vi "test.vi"() -> ()   [LabVIEW 2014]
panel:
  in  "id 4":string="R-6"
  in  "new_setting 4":dbl=0.2
  in  "id 3":string="R-6"
  in  "new_setting 3":dbl=1.0
  in  "new_setting 2":dbl=1.0
  in  "id 2":string="R-5"
  in  "new_setting":dbl=0.2
  in  "id":string="R-5"
  in  "Attribute 3":i32(ring)=201 items=["Depth"=200, "Volume"=201, "Flow"=202, "Setting"=203, "Froude"=204, "Inflow"=205, "Flooding"=206, "Precipitation"=207, "Runoff"=208]
  in  "Unit system 3":i32(ring)=1 items=["US", "SI"]
  in  "object_id 3":string="V-3"
  in  "object_id 2":string="V-2"
  in  "Attribute 2":i32(ring)=201 items=["Depth"=200, "Volume"=201, "Flow"=202, "Setting"=203, "Froude"=204, "Inflow"=205, "Flooding"=206, "Precipitation"=207, "Runoff"=208]
  in  "Unit system 2":i32(ring)=1 items=["US", "SI"]
  out "Graph":dbl[][](graph)
  in  "Path":path=path "C:/Users/andres riaño/Dropbox/Proyecto Aguas/Software/MatSWMM/MatSWMM 5.1.009/LabVIEW module/x64/swmm_files/3tanks.INP"
  in  "Unit system":i32(ring)=1 items=["US", "SI"]
  in  "Attribute":i32(ring)=201 items=["Depth"=200, "Volume"=201, "Flow"=202, "Setting"=203, "Froude"=204, "Inflow"=205, "Flooding"=206, "Precipitation"=207, "Runoff"=208]
  in  "object_id":string="V-1"
  # "If the volume of V-3 exceeds 4000m3/s"
  # "If the volume of V-2 exceeds 9000m3/s"
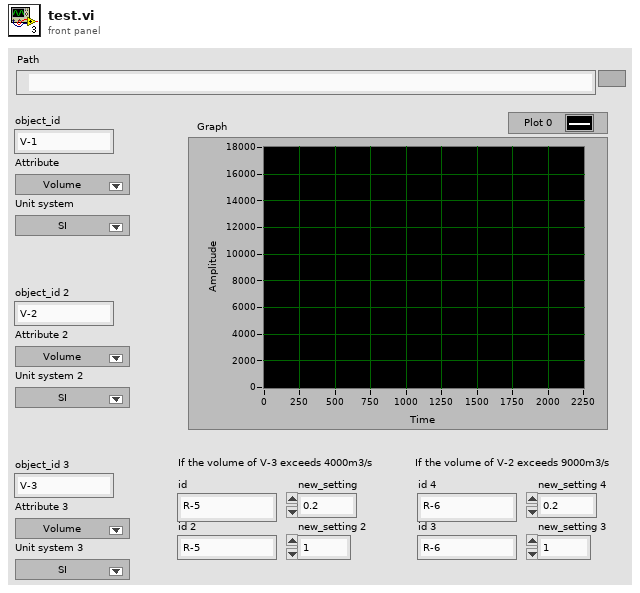
[diagram p1: front panel]
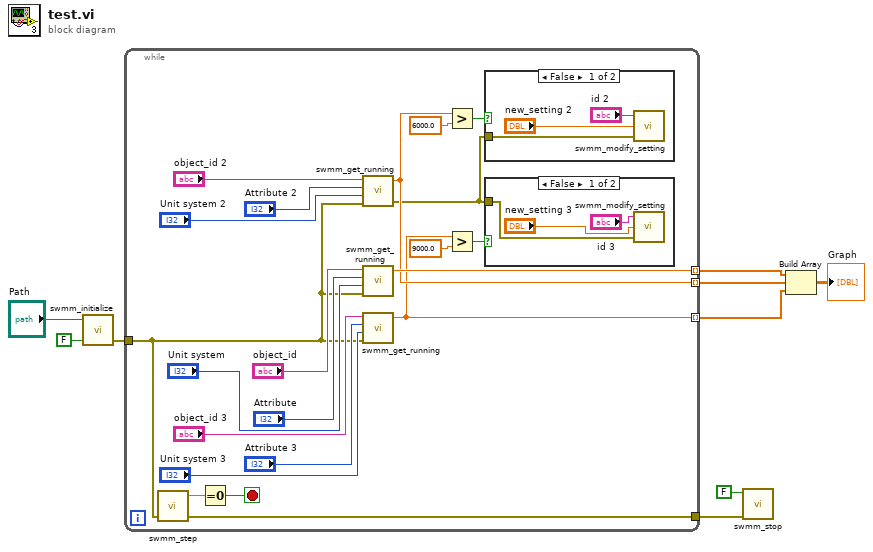
[diagram p0: block diagram]
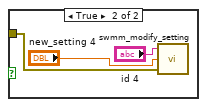
[diagram p2: hidden frame]
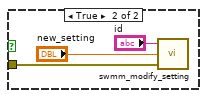
[diagram p3: hidden frame]
diagram:
  n1 = call "swmm_initialize.vi"("Success msg?"=FALSE, "SWMM Input File (.inp)"="Path") -> ("error out"=w8:errorcluster)  [unwired: 3 in]
  n2 = while {
    tunnel: [w25] -> w9
    tunnel: w8 -> [w18]
    tunnel: [w14] -> w4 mode=indexing
    tunnel: [w15] -> w5 mode=indexing
    tunnel: [w11] -> w3 mode=indexing
    stop <- w30 stop-if-true
    n3 = call "swmm_step.vi"("error in (no error)"=w18) -> ("error out"=w25:errorcluster, "new_elapsed_time"=w29:dbl)  [unwired: 3 in]
    n4 = Equal To 0?(x=w29) -> (x = 0?=w30:bool)
    n5 = call "swmm_get_running.vi"("error in"=w18, "Unit system"="Unit system 2", "Attribute"="Attribute 2", "object_id"="object_id 2") -> ("error out"=w10:errorcluster, "value"=w14:dbl)  [unwired: 1 in]
    n6 = call "swmm_get_running.vi"("error in"=w18, "Unit system"="Unit system", "Attribute"="Attribute", "object_id"="object_id") -> ("value"=w15:dbl)  [unwired: 1 in, 1 out]
    n7 = call "swmm_get_running.vi"("error in"=w18, "Unit system"="Unit system 3", "Attribute"="Attribute 3", "object_id"="object_id 3") -> ("value"=w11:dbl)  [unwired: 1 in, 1 out]
    n8 = Greater?(x=w14, y=6000.0) -> (0:w16:bool)
    n9 = Greater?(x=w11, y=9000.0) -> (0:w13:bool)
    n10 = case shown="False" w16 {
      tunnel: w10 -> [w37 w40]
      frame False {
        n11 = call "swmm_modify_setting.vi"("error in"=w37, "new_setting"="new_setting 2", "id"="id 2") -> ()  [unwired: 1 in, 2 out]
      }
      frame True {
        n12 = call "swmm_modify_setting.vi"("error in"=w40, "new_setting"="new_setting", "id"="id") -> ()  [unwired: 1 in, 2 out]
      }
    }
    n13 = case shown="False" w13 {
      tunnel: w10 -> [w31 w34]
      frame False {
        n14 = call "swmm_modify_setting.vi"("error in"=w31, "new_setting"="new_setting 3", "id"="id 3") -> ()  [unwired: 1 in, 2 out]
      }
      frame True {
        n15 = call "swmm_modify_setting.vi"("error in"=w34, "new_setting"="new_setting 4", "id"="id 4") -> ()  [unwired: 1 in, 2 out]
      }
    }
  }
  n16 = call "swmm_stop.vi"("error in"=w9, "Success msg?"=FALSE) -> ()  [unwired: 2 in, 4 out]
  n17 = Build Array(w5, w4, w3) -> (→"Graph":dbl[][])
